vi "LabelToControl.vi"(11 "ControlName":string) -> (3 "String":string)   [LabVIEW 2015]
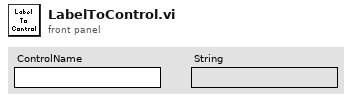
[diagram p1: front panel]
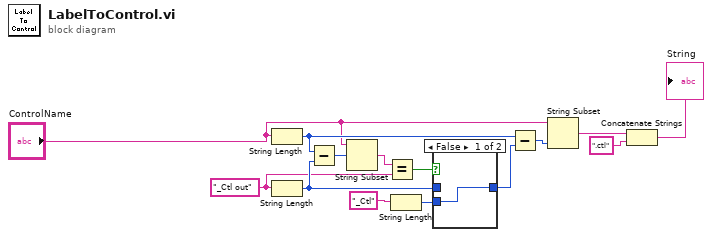
[diagram p0: block diagram]
diagram:
  w10 = "_Ctl out"
  n1 = String Length(string="ControlName") -> (length=w7:i32)
  n2 = String Length(string=w10) -> (length=w12:i32)
  n3 = Subtract(x=w7, y=w12) -> (x-y=w8:i32)
  n4 = String Subset(string="ControlName", offset (0)=w8) -> (substring=w9:string)  [unwired: 1 in]
  n5 = Equal?(x=w9, y=w10) -> (x = y?=w11:bool)
  n6 = String Length(string="_Ctl") -> (length=w13:i32)
  n7 = case shown="False" w11 {
    tunnel: w12 -> [_ w16]
    tunnel: w13 -> [w15 _]
    tunnel: [w15 w16] -> w14
    frame False {
    }
    frame True {
    }
  }
  n8 = Subtract(x=w7, y=w14) -> (x-y=w1:i32)
  n9 = String Subset(string="ControlName", length (rest)=w1) -> (substring=w2:string)  [unwired: 1 in]
  n10 = Concatenate Strings(w2, ".ctl" ("string")) -> (→"String":string)
